vi "Close Stream.vi"(0 "video in":refnum<class "MSC Video.lvclass">, 5 "error in (no error)":errorcluster) -> (14 "video out":refnum<class "MSC Video.lvclass">, 19 "error out":errorcluster)   [LabVIEW 2014, in "MSC Video.lvclass"]
doc: "Closes an opened stream. This vi works with all kinds of streams provided by this library.\nUse this function to free the resource."
uses:
  MSC Video.lvclass
  MSC Video.lvclass/MSC Video.ctl
  Dependencies/x86/MSC I Process32.dll
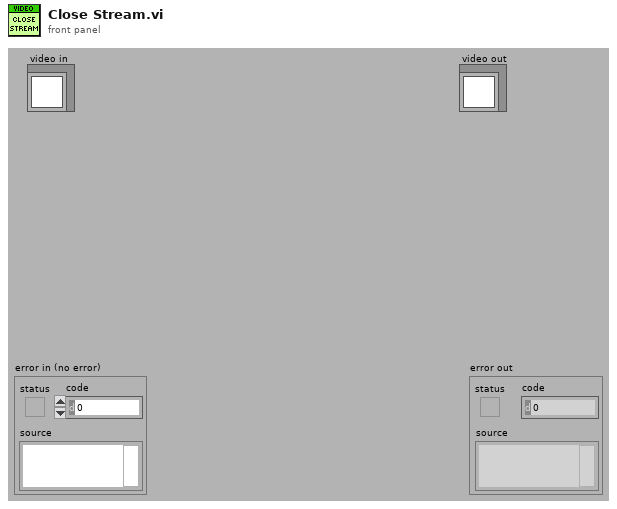
[diagram p1: front panel]
types:
  T1 = typedef "MSC Video.lvclass/Video.ctl" = cluster{"Pointer":u64, "CamID":i32, "File Path":path, "Network Address":string, "opened":bool}
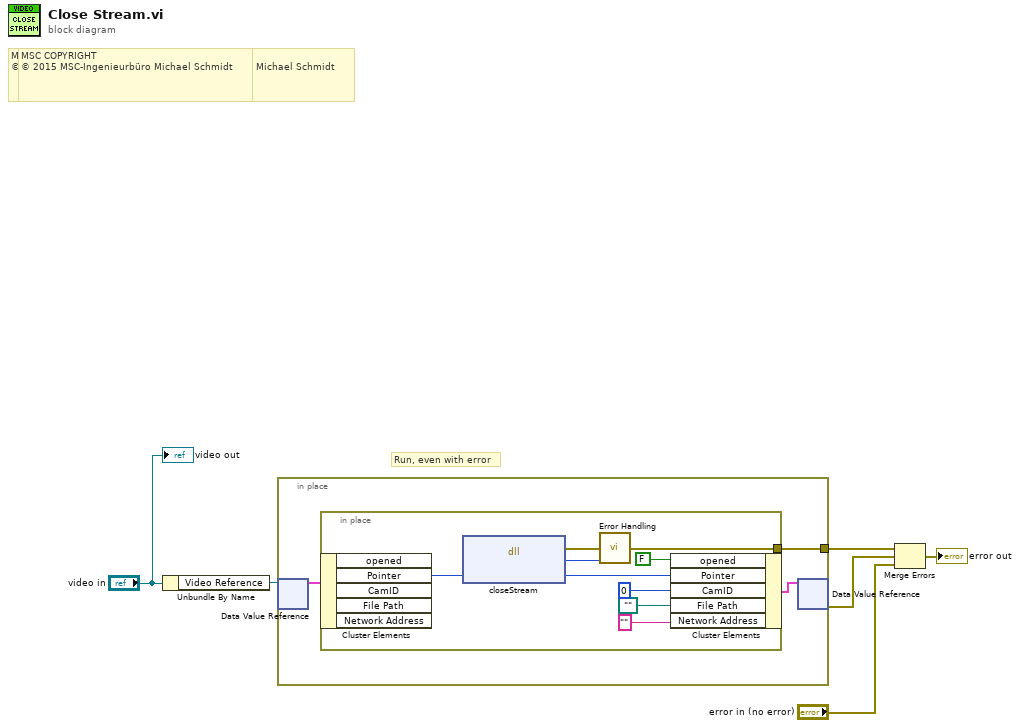
[diagram p0: block diagram]
diagram:
  # "MSC COPYRIGHT\n© 2016 MSC-Ingenieurbüro Michael Schmidt"
  # "MSC COPYRIGHT\n© 2016 MSC-Ingenieurbüro Michael Schmidt"
  # "MSC COPYRIGHT\n© 2015 MSC-Ingenieurbüro Michael Schmidt"
  # "Run, even with error"
  n1 = Unbundle By Name("video in") -> ("Video Reference"=w5:refnum<data-value>)
  n2 = in-place {
    in-place-border: [w7] -> w4
    n3 = in-place-dvr #1(w5) -> (w8:T1)  [unwired: 1 out]
    n4 = in-place {
      in-place-border: [w14] -> w7
      n5 = in-place-cluster #2(w8) -> ("Pointer"=w18:u64)  [unwired: 4 out]
      n6 = dll-call lib="C:/Users/MSC/LabVIEW Projekte/LV 2014/MSC I-Process/user.lib/MSC-I Process/Dependencies/x86/MSC I Process*.dll" fn="closeStream"("pointer"=w18) -> (error out=w16:errorcluster, "error"=w15:i32, "pointer"=w17:u64)  [unwired: 3 in, 1 out]
      n7 = call "Error Handling.vi"("error in (no error)"=w16, "return type"=w15) -> ("error out"=w14:errorcluster)  [unwired: 12 in, 1 out]
      n8 = in-place-cluster #2("opened"=FALSE, "Pointer"=w17, "CamID"=0, "File Path"=path "", "Network Address"="") -> (w9:T1)
    }
    n9 = in-place-dvr #1(w9) -> (w3:errorcluster)  [unwired: 1 out]
  }
  n10 = Merge Errors(w4, w3, "error in (no error)") -> (→"error out":errorcluster)
  "video out" <- "video in"
